vi "LOGIN.vi"() -> ()   [LabVIEW 2017]
uses:
  GLOBAL/auto.vi
  <vilib>/addons/database/Connection.llb/DB Tools Open Connec (Path).vi
  <vilib>/addons/database/NI_Database_API.lvlib
panel:
  out "PASSWORD":string[](array[string])
  out "ATHOR":string[](array[string])
  out "USER":string[](array[string])
  in  "error in":errorcluster
  in  "Cancel":bool
  in  "OK":bool
  in  "USER NAME":string(combo)
  in  "PASSWORD":string
  # "LOGIN"
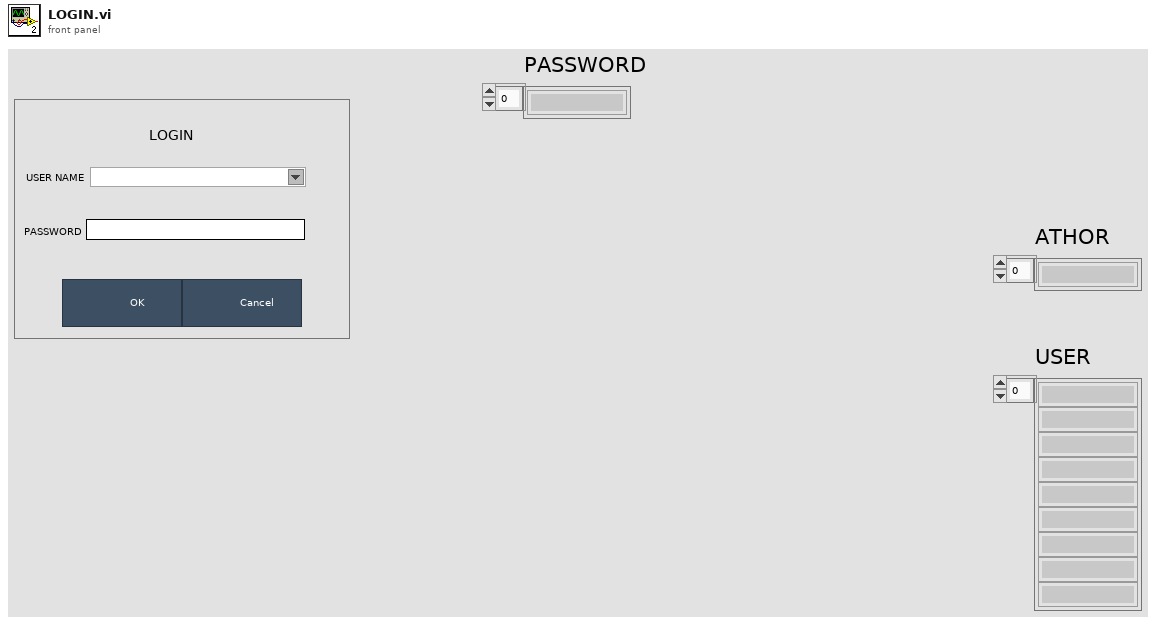
[diagram p1: front panel]
types:
  T1 = typedef "NI_Database_API.lvlib/Conn ObjectReference.ctl" = refnum<k1>
  T2 = enum32{"invalid app kind", "Development System", "Run Time System", "Student Edition", "Embedded LabVIEW", "Evaluation", "Custom"}
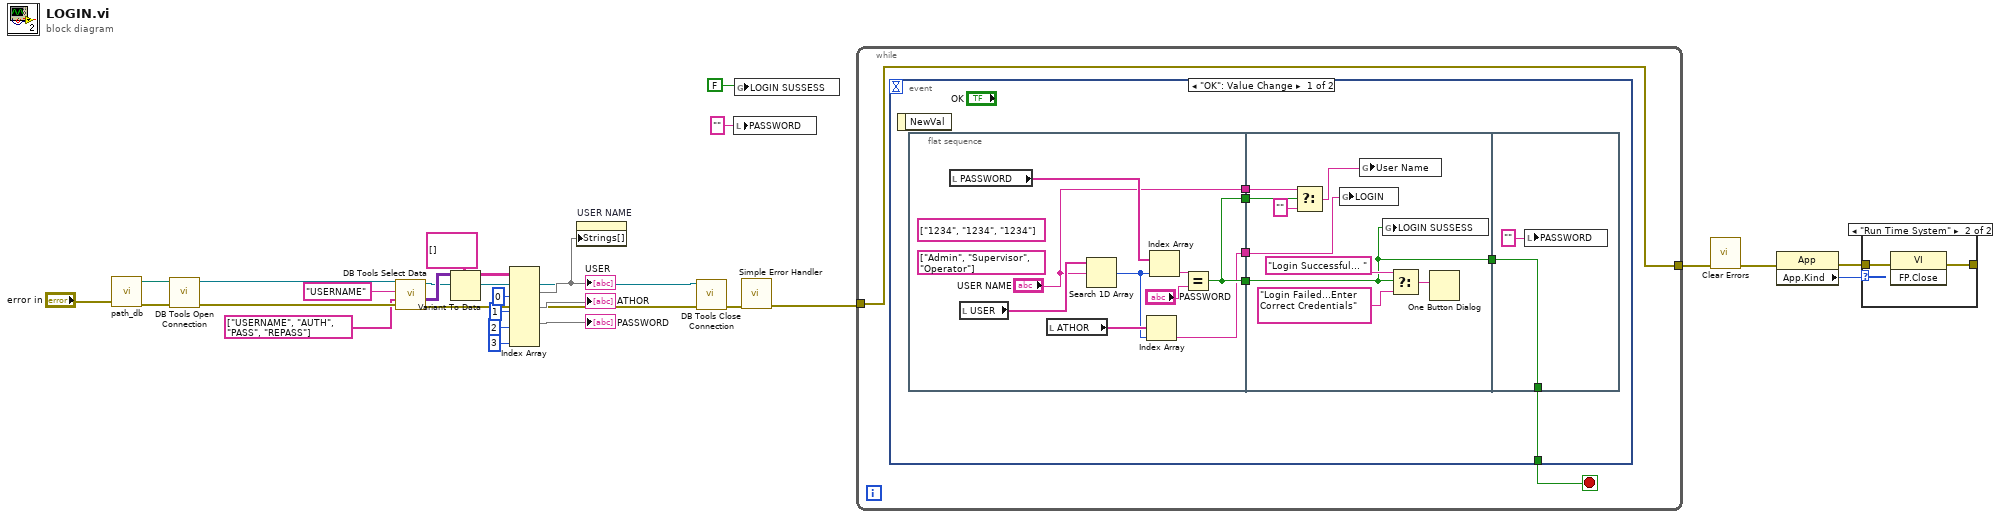
[diagram p0: block diagram]
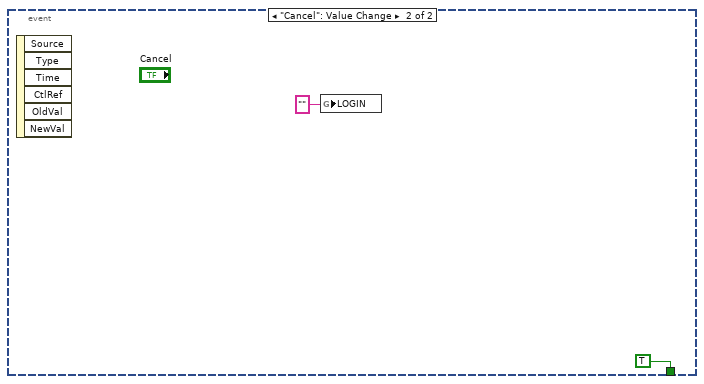
[diagram p3: hidden frame]
diagram:
  n1 = call "path_db.vi"("error in"="error in") -> ("error out"=w5:errorcluster, "resulting string"=w4:path)  [unwired: 9 in]
  n2 = call-poly <vilib>:"DB Tools Open Connection.vi"("error in (no error)"=w5, "connection information"=w4) -> ("error out"=w17:errorcluster, "connection reference"=w18:T1)  [unwired: 6 in]
  n3 = call <vilib>:"DB Tools Select Data.vi"("error in (no error)"=w17, "columns"=string[] ["USERNAME", "AUTH", "PASS", "REPASS"], "table"="USERNAME", "connection reference"=w18) -> ("error out"=w8:errorcluster, "data"=w22:variant[][], "connection reference out"=w6:T1)  [unwired: 2 in]
  n4 = Variant To Data(type=string[][] [], Variant=w22) -> (data=w19:string[][])  [unwired: 1 in, 1 out]
  n5 = Index Array(array=w19, index (col) #1=0 ("disabled index (col)"), index (col) #2=1 ("index (col)"), index (col) #3=2 ("index (col)"), index (col) #4=3 ("index (col)")) -> (element #1=w10:string[], element #2=→"ATHOR":string[], element #3=→"PASSWORD":string[])  [unwired: 4 in, 1 out]
  "USER" <- w10
  n6 = property on="USER NAME" class="CmbBox"("Strings[]"=w10) -> ()  [unwired: 2 in, 2 out]
  n7 = call <vilib>:"DB Tools Close Connection.vi"("error in (no error)"=w8, "connection reference"=w6) -> ("error out"=w9:errorcluster)  [unwired: 5 in]
  n8 = local write "PASSWORD"("" ("PASSWORD")) -> ()
  n9 = global write "auto.vi" "LOGIN SUSSESS"(FALSE ("Login Success")) -> ()
  n10 = call <vilib>:"Simple Error Handler.vi"("error in (no error)"=w9) -> ("error out"=w7:errorcluster)  [unwired: 4 in, 4 out]
  n11 = while {
    tunnel: [w28] -> w1
    tunnel: w7 -> [w28]
    stop <- w29 stop-if-true
    n12 = event shown="[0] \"OK\": Value Change" {
      selector: _ -> [_ _]
      dyn-events: _ -> [_ _]
      timeout: _ -> [_ _]
      tunnel: [w33 TRUE] -> w29
      event "OK": Value Change {
        n13 = event-data() -> ()  [unwired: 1 in, 1 out]
        n14 = flat-sequence {
          tunnel: [w42] -> w35
          tunnel: [w42] -> w32
          tunnel: ["USER NAME"] -> w31
          tunnel: [w38] -> w30
          tunnel: w35 -> [w47]
          tunnel: [w47] -> w34
          tunnel: w32 -> [w50]
          tunnel: w31 -> [w49]
          tunnel: w30 -> [w46]
          tunnel: w34 -> [w55]
          tunnel: [w55] -> w33
          frame #0 {
            (unwired) string[] ["1234", "1234", "1234"]
            (unwired) string[] ["Admin", "Supervisor", "Operator"]
            n15 = local read "PASSWORD"() -> (w41:string[])
            n16 = local read "USER"() -> (w37:string[])
            n17 = local read "ATHOR"() -> (w40:string[])
            n18 = Search 1D Array(1D array=w37, element="USER NAME") -> (index of element=w39:i32)  [unwired: 1 in]
            n19 = Index Array(array=w40, index=w39) -> (element=w38:string)
            n20 = Index Array(array=w41, index=w39) -> (element=w44:string)
            n21 = Equal?(x=w44, y="PASSWORD") -> (x = y?=w42:bool)
          }
          frame #1 {
            n22 = Select(t=w49, s=w50, f="") -> (s? t:f=w45:string)
            n23 = global write "auto.vi" "LOGIN"(w46) -> ()
            n24 = global write "auto.vi" "User Name"(w45) -> ()
            n25 = global write "auto.vi" "LOGIN SUSSESS"(w47) -> ()
            n26 = Select(t="Login Successful... " ("message"), s=w47, f="Login Failed...Enter Correct Credentials" ("message")) -> (s? t:f=w51:string)
            n27 = One Button Dialog(message=w51) -> ()  [unwired: 1 in, 1 out]
          }
          frame #2 {
            n28 = local write "PASSWORD"("" ("PASSWORD")) -> ()
          }
        }
      }
      event "Cancel": Value Change {
        n29 = event-data() -> ()  [unwired: 1 in, 6 out]
        n30 = global write "auto.vi" "LOGIN"("" ("Login")) -> ()
      }
    }
  }
  n31 = call <vilib>:"Clear Errors.vi"("error in (no error)"=w1) -> ("error out"=w2:errorcluster)  [unwired: 5 in, 1 out]
  n32 = property class="App"(error in=w2) -> (error out=w25:errorcluster, "App.Kind"=w26:T2)  [unwired: 1 in, 1 out]
  n33 = case shown="\"Run Time System\"" w26 {
    tunnel: w25 -> [w58 w60]
    tunnel: [w58 w59] -> _
    frame Default {
    }
    frame "Run Time System" {
      n34 = invoke class="VI" method="FP.Close"(error in=w60) -> (error out=w59:errorcluster)  [unwired: 2 in, 2 out]
    }
  }
